vi "settings.vi"(0 "task":string, 1 "blocksPerDay":string, 2 "hand":string, 3 "procedure":string, 4 "trialsPerBlock":string, 6 "targets_array":string, 7 "LabVIEW Web Service Request":refnum<class "Web Request.lvclass">, 8 "fixationPeriod":string, 9 "level":string, 10 "date":string, 11 "mode":string) -> (5 "progress":string)   [LabVIEW 2020]
uses:
  <vilib>/wsapi/Web Request.lvclass
  Global 1.vi
panel:
  # "Use the Web Service Request input terminal to call the VIs on the Web Services palette. Do not remove it from the connector pane unless you don't need access to the palette."
  # "Each additional control wired to the connector pane will be available as an input in the URL. To include an indicator in terminal-mode output (the default setting), it must also be wired to the connector pane."
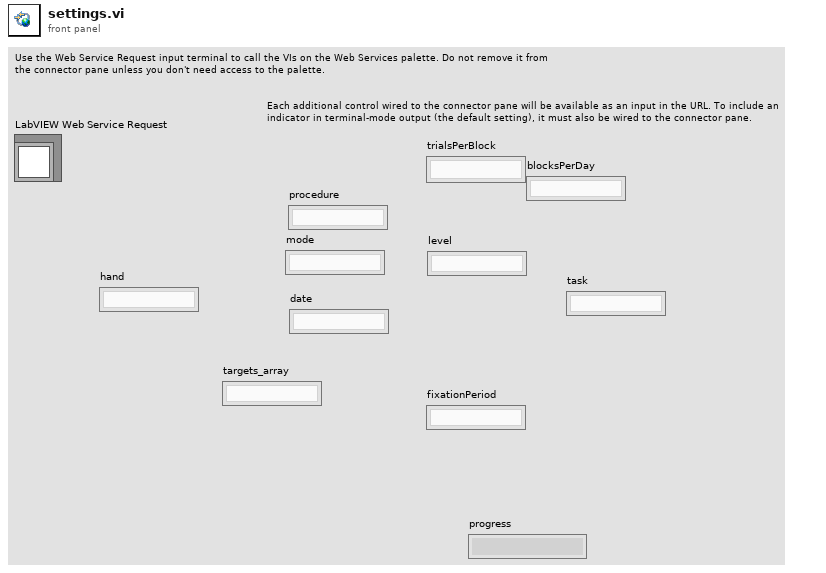
[diagram p1: front panel]
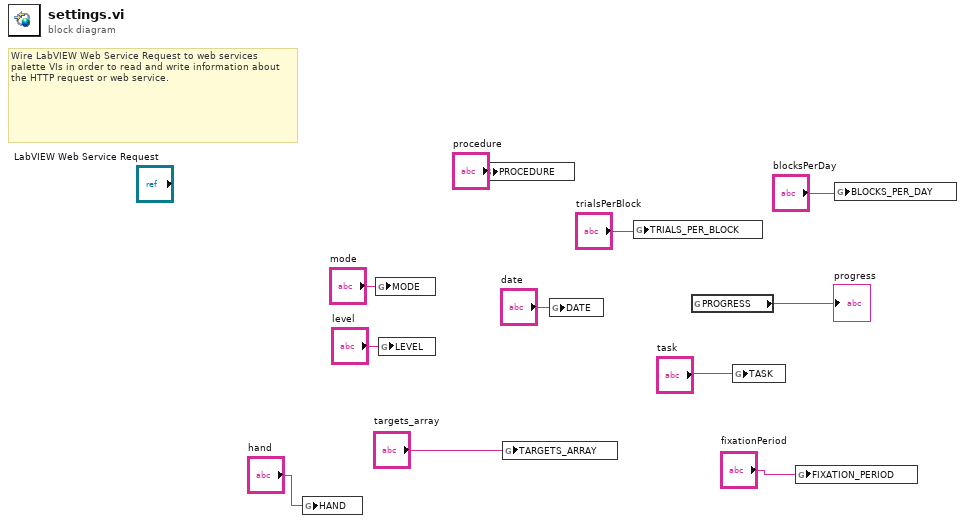
[diagram p0: block diagram]
diagram:
  # "Wire LabVIEW Web Service Request to web services palette VIs in order to read and write information about the HTTP request or web service."
  n1 = global write "Global 1.vi" "HAND"("hand") -> ()
  n2 = global write "Global 1.vi" "MODE"("mode") -> ()
  n3 = global write "Global 1.vi" "LEVEL"("level") -> ()
  n4 = global write "Global 1.vi" "PROCEDURE"("procedure") -> ()
  n5 = global write "Global 1.vi" "TARGETS_ARRAY"("targets_array") -> ()
  n6 = global write "Global 1.vi" "DATE"("date") -> ()
  n7 = global write "Global 1.vi" "TRIALS_PER_BLOCK"("trialsPerBlock") -> ()
  n8 = global read "Global 1.vi" "PROGRESS"() -> (→"progress":string)
  n9 = global write "Global 1.vi" "TASK"("task") -> ()
  n10 = global write "Global 1.vi" "FIXATION_PERIOD"("fixationPeriod") -> ()
  n11 = global write "Global 1.vi" "BLOCKS_PER_DAY"("blocksPerDay") -> ()
